vi "Write Network Interface.vi"(8 "error in (no error)":errorcluster, 10 "Network Interface":refnum<class "Network Interface.lvclass">, 11 "Transmission Data Unit in":refnum<class "Transmission Data Unit.lvclass">) -> (0 "error out":errorcluster, 3 "Transmission Data Unit out":refnum<class "Transmission Data Unit.lvclass">)   [LabVIEW 2021, in "Transmission Data Unit.lvclass"]
uses:
  Transmission Data Unit.lvclass
  Transmission Data Unit.lvclass/Transmission Data Unit.ctl
  Network Interface/Network Interface.lvclass
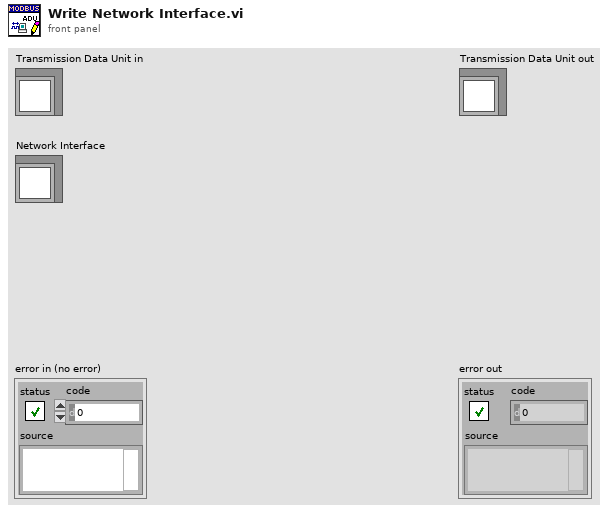
[diagram p1: front panel]
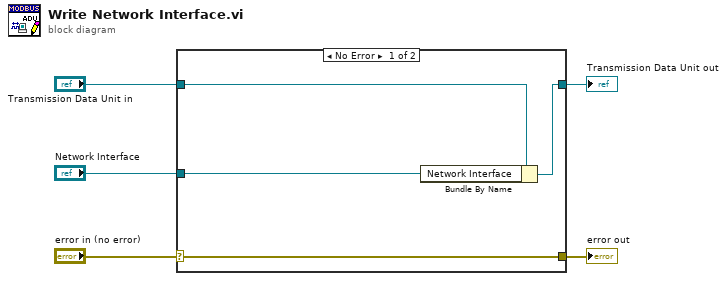
[diagram p0: block diagram]
diagram:
  n1 = case shown="No Error" "error in (no error)" {
    selector: "error in (no error)" -> [w9 w10]
    tunnel: [w9 w10] -> w4
    tunnel: [w7 w11] -> w2
    tunnel: "Transmission Data Unit in" -> [w8 w11]
    tunnel: "Network Interface" -> [w6 _]
    frame No Error {
      n2 = Bundle By Name(cluster=w8, "Network Interface"=w6) -> (w7:refnum<class "Transmission Data Unit.lvclass">)
    }
    frame Error {
    }
  }
  "error out" <- w4
  "Transmission Data Unit out" <- w2
